vi "pack_item.vi"(3 "error in":errorcluster, 4 "x":variant, 5 "p":u64) -> (0 "error out":errorcluster, 2 "p out":u64)   [LabVIEW 2019, in "msgpack.lvlib"]
doc: "Packs an object into the msgpack buffer. All types supported by msgpack are compatible.\n\nSupported types are\n- numeric types (integers, floats)\n- arrays of numeric types\n- boolean\n- clusters\n- strings (raw data)\n- void variants (packed as null)"
uses:
  msgpack.lvlib
  <vilib>/Utility/VariantDataType/VariantType.lvlib
  msgpackalt.dll
panel:
  # "msgpack"
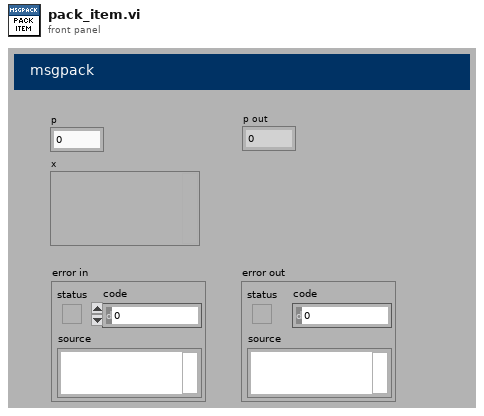
[diagram p1: front panel]
types:
  T1 = typedef "VariantType.lvlib/Type.ctl" = enum8{"Invalid Type", "Void", "I8", "I16", "I32", "I64", "U8", "U16", "U32", "U64", "Single Float", "Double Float", "Extended Float", "Single Complex", "Double Complex", "Extended Complex", "Enum U8", "Enum U16", "Enum U32", "Enum U64", "Single Float With Unit", "Double Float With Unit", "Extended Float With Unit", "Single Complex with Unit", "Double Complex with Unit", "Extended Complex with Unit", "Boolean", "String", "Path", "Picture", "Tag", "Array", "Cluster", "Variant", "LV Variant", "Waveform", "Timestamp", "Digital Waveform", "Digital Data", "ExpressData", "Refnum", "External Data", "VI", "Poly VI", "LabVIEW Class Instance", "Fixed Point"}
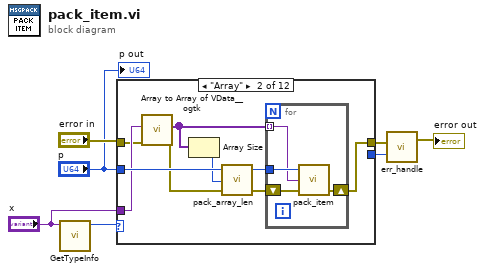
[diagram p0: block diagram]
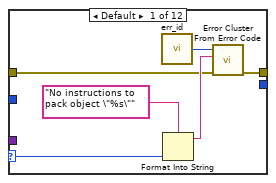
[diagram p2: hidden frame]
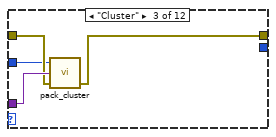
[diagram p3: hidden frame]
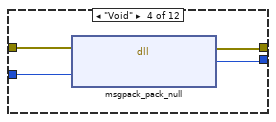
[diagram p4: hidden frame]
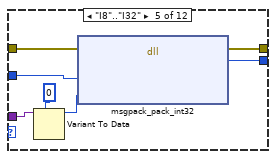
[diagram p5: hidden frame]
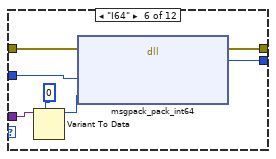
[diagram p6: hidden frame]
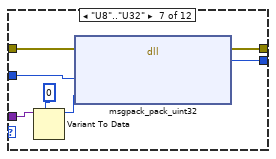
[diagram p7: hidden frame]
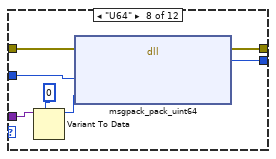
[diagram p8: hidden frame]
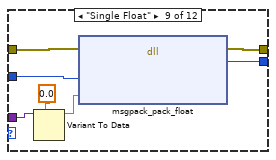
[diagram p9: hidden frame]
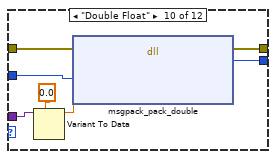
[diagram p10: hidden frame]
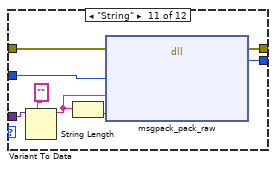
[diagram p11: hidden frame]
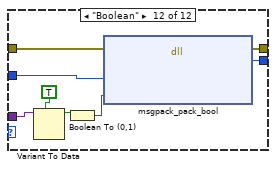
[diagram p12: hidden frame]
diagram:
  n1 = call <vilib>:"GetTypeInfo.vi"("Variant"="x") -> ("Type Enum"=w5:T1)  [unwired: 6 in, 4 out]
  n2 = case shown="\"Array\"" w5 {
    selector: w5 -> [w8 _ _ _ _ _ _ _ _ _ _ _]
    tunnel: "error in" -> [w9 w20 w29 w34 w41 w48 w55 w62 w69 w76 w84 w92]
    tunnel: [w10 w14 w28 w32 w40 w47 w54 w61 w68 w75 w83 w91] -> w3
    tunnel: "p" -> [_ w22 w27 w33 w39 w46 w53 w60 w67 w74 w82 w90]
    tunnel: "x" -> [_ w21 w30 _ w38 w45 w52 w59 w66 w73 w81 w89]
    tunnel: [_ _ _ w31 w35 w42 w49 w56 w63 w70 w77 w85] -> w1
    frame Default {
      n3 = call "err_id.vi"() -> ("error code"=w11:i32)
      n4 = Format Into String(format string="No instructions to pack object \"%s\"", w8) -> (resulting string=w13:string)  [unwired: 2 in, 1 out]
      n5 = call <vilib>:"Error Cluster From Error Code.vi"("error in (no error)"=w9, "error message (\"\")"=w13, "error code (0)"=w11) -> ("error out"=w10:errorcluster)  [unwired: 6 in]
    }
    frame "Array" {
      n6 = call "Array to Array of VData__ogtk.vi"("error in (no error)"=w20, "MultiD Array"=w21) -> ("error out"=w18:errorcluster, "1D Array of Variants"=w15:variant[])  [unwired: 8 in]
      n7 = Array Size(array=w15) -> (size(s)=w19:i32)
      n8 = call "pack_array_len.vi"("error in"=w18, "n"=w19, "p"=w22) -> ("error out"=w17:errorcluster, "p out"=w16:u64)  [unwired: 1 in]
      n9 = for {
        shift-right: [w23] -> w14
        shift-left: w17 -> [w26]
        tunnel: w16 -> [w25]
        tunnel: w15 -> [w24] mode=indexing
        n10 = call "pack_item.vi"("error in"=w26, "x"=w24, "p"=w25) -> ("error out"=w23:errorcluster)  [unwired: 1 in, 1 out]
      }
    }
    frame "Cluster" {
      n11 = call "pack_cluster.vi"("error in"=w29, "cluster"=w30, "p"=w27) -> ("error out"=w28:errorcluster)  [unwired: 1 in, 1 out]
    }
    frame "Void" {
      n12 = dll-call lib="C:/Users/Patrick/Documents/GitHub/Instrument-Framework/lvsrc/SMOs/JSON-RPC-2019/lv-venv/lv.lib/vi.lib/addons/msgpack/msgpackalt.dll" fn="msgpack_pack_null"(error in=w34, "p"=w33) -> (error out=w32:errorcluster, "return type"=w31:i32)  [unwired: 3 in, 1 out]
    }
    frame "I8".."I32" {
      n13 = Variant To Data(type=0, Variant=w38) -> (data=w36:i32)  [unwired: 1 in, 1 out]
      n14 = dll-call lib="C:/Users/Patrick/Documents/GitHub/Instrument-Framework/lvsrc/SMOs/JSON-RPC-2019/lv-venv/lv.lib/vi.lib/addons/msgpack/msgpackalt.dll" fn="msgpack_pack_int32"(error in=w41, "p"=w39, "x"=w36) -> (error out=w40:errorcluster, "return type"=w35:i32)  [unwired: 4 in, 1 out]
    }
    frame "I64" {
      n15 = Variant To Data(type=i64 0, Variant=w45) -> (data=w43:i64)  [unwired: 1 in, 1 out]
      n16 = dll-call lib="C:/Users/Patrick/Documents/GitHub/Instrument-Framework/lvsrc/SMOs/JSON-RPC-2019/lv-venv/lv.lib/vi.lib/addons/msgpack/msgpackalt.dll" fn="msgpack_pack_int64"(error in=w48, "p"=w46, "x"=w43) -> (error out=w47:errorcluster, "return type"=w42:i32)  [unwired: 4 in, 1 out]
    }
    frame "U8".."U32" {
      n17 = Variant To Data(type=u32 0, Variant=w52) -> (data=w50:u32)  [unwired: 1 in, 1 out]
      n18 = dll-call lib="C:/Users/Patrick/Documents/GitHub/Instrument-Framework/lvsrc/SMOs/JSON-RPC-2019/lv-venv/lv.lib/vi.lib/addons/msgpack/msgpackalt.dll" fn="msgpack_pack_uint32"(error in=w55, "p"=w53, "x"=w50) -> (error out=w54:errorcluster, "return type"=w49:i32)  [unwired: 4 in, 1 out]
    }
    frame "U64" {
      n19 = Variant To Data(type=u64 0, Variant=w59) -> (data=w57:u64)  [unwired: 1 in, 1 out]
      n20 = dll-call lib="C:/Users/Patrick/Documents/GitHub/Instrument-Framework/lvsrc/SMOs/JSON-RPC-2019/lv-venv/lv.lib/vi.lib/addons/msgpack/msgpackalt.dll" fn="msgpack_pack_uint64"(error in=w62, "p"=w60, "x"=w57) -> (error out=w61:errorcluster, "return type"=w56:i32)  [unwired: 4 in, 1 out]
    }
    frame "Single Float" {
      n21 = Variant To Data(type=sgl 0.0, Variant=w66) -> (data=w64:sgl)  [unwired: 1 in, 1 out]
      n22 = dll-call lib="C:/Users/Patrick/Documents/GitHub/Instrument-Framework/lvsrc/SMOs/JSON-RPC-2019/lv-venv/lv.lib/vi.lib/addons/msgpack/msgpackalt.dll" fn="msgpack_pack_float"(error in=w69, "p"=w67, "x"=w64) -> (error out=w68:errorcluster, "return type"=w63:i32)  [unwired: 4 in, 1 out]
    }
    frame "Double Float" {
      n23 = Variant To Data(type=0.0, Variant=w73) -> (data=w71:dbl)  [unwired: 1 in, 1 out]
      n24 = dll-call lib="C:/Users/Patrick/Documents/GitHub/Instrument-Framework/lvsrc/SMOs/JSON-RPC-2019/lv-venv/lv.lib/vi.lib/addons/msgpack/msgpackalt.dll" fn="msgpack_pack_double"(error in=w76, "p"=w74, "x"=w71) -> (error out=w75:errorcluster, "return type"=w70:i32)  [unwired: 4 in, 1 out]
    }
    frame "String" {
      n25 = Variant To Data(type="", Variant=w81) -> (data=w79:string)  [unwired: 1 in, 1 out]
      n26 = String Length(string=w79) -> (length=w78:i32)
      n27 = dll-call lib="C:/Users/Patrick/Documents/GitHub/Instrument-Framework/lvsrc/SMOs/JSON-RPC-2019/lv-venv/lv.lib/vi.lib/addons/msgpack/msgpackalt.dll" fn="msgpack_pack_raw"(error in=w84, "p"=w82, "x"=w79, "n"=w78) -> (error out=w83:errorcluster, "return type"=w77:i32)  [unwired: 5 in, 1 out]
    }
    frame "Boolean" {
      n28 = Variant To Data(type=TRUE, Variant=w89) -> (data=w87:bool)  [unwired: 1 in, 1 out]
      n29 = Boolean To (0,1)(Boolean=w87) -> (0, 1=w86:i16)
      n30 = dll-call lib="C:/Users/Patrick/Documents/GitHub/Instrument-Framework/lvsrc/SMOs/JSON-RPC-2019/lv-venv/lv.lib/vi.lib/addons/msgpack/msgpackalt.dll" fn="msgpack_pack_bool"(error in=w92, "p"=w90, "x"=w86) -> (error out=w91:errorcluster, "return type"=w85:i32)  [unwired: 4 in, 1 out]
    }
  }
  n31 = call "err_handle.vi"("retval"=w1, "error in"=w3) -> ("error out"=→"error out":errorcluster)  [unwired: 1 in]
  "p out" <- "p"
